vi "Matrix_Replace_Sub_array.vi"(8 "Vector":dbl[](array[numeric]), 9 "Index Column":i32, 10 "Index Row":i32, 11 "Array":dbl[][](array[numeric])) -> (3 "New Array":dbl[][](array[numeric]))   [LabVIEW 2019, in "Trajectory_Library.lvlib"]
doc: "This VI is used to replace an array inside a matrix where the array has a smaller size than the rows of the matrix.\n\nCreated by Davis Montenegro\n10-05-2013"
uses:
  Trajectory_Library.lvlib
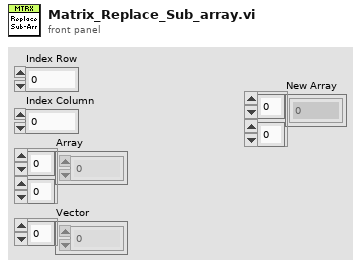
[diagram p1: front panel]
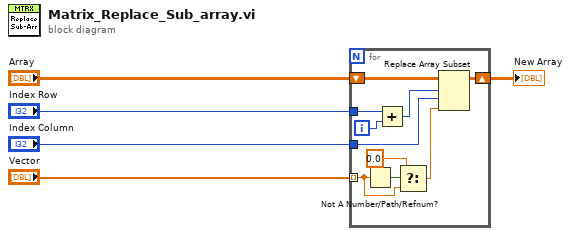
[diagram p0: block diagram]
diagram:
  n1 = for {
    shift-right: [w15] -> w5
    shift-left: "Array" -> [w14]
    tunnel: "Vector" -> [w7] mode=indexing
    tunnel: "Index Column" -> [w13]
    tunnel: "Index Row" -> [w11]
    i -> [w12]
    n2 = Not A Number/Path/Refnum?(number/path/refnum=w7) -> (NaN/Path/Refnum?=w8:bool)
    n3 = Add(x=w11, y=w12) -> (x+y=w10:i32)
    n4 = Select(t=0.0, s=w8, f=w7) -> (s? t:f=w6:dbl)
    n5 = Replace Array Subset(array=w14, new element=w6, index (row)=w10, index (col)=w13) -> (w15:dbl[][])
  }
  "New Array" <- w5
